vi "Read-Humidity.vi"(7 "Slave Address (7-bit)":u8 format="%x", 8 "error in (no error)":errorcluster, 9 "T_fine":dbl, 10 "Comp Coeffs":T1 {"dig_H6" format="%0d"; "dig_H5" format="%0d"; "dig_H4" format="%0d"; "dig_H3" format="%0d"; "dig_H2" format="%0d"; "dig_H1" format="%0d"; "dig_P9" format="%0d"; "dig_P8" format="%0d"; "dig_P7" format="%0d"; "dig_P6" format="%0d"; "dig_P5" format="%0d"; "dig_P4" format="%0d"; "dig_P3" format="%0d"; "dig_P2" format="%0d"; "dig_P1" format="%0d"; "dig_T3" format="%0d"; "dig_T2" format="%0d"; "dig_T1" format="%0d"}, 11 "I2C Ref In":T2) -> (0 "error out":errorcluster, 3 "I2C Ref Out":T2={"myRIO Reference"={"myRIO Model"=enum."Unknown", "myRIO Hardware Reference"={"Generic FPGA Reference"=refnum, "Allow multiple opens"=FALSE}}, "I2C Channels Enum"=enum."Not Connected", "I2C Configuration"={"I2C Transfer Rate"=enum."Fast mode (400 kbps)"}}, 4 "ADC RAW HUMIDITY":u32, 5 "Bytes Read":u8[](array[numeric]), 6 "Humidity":dbl)   [LabVIEW 2015]
uses:
  <vilib>/myRIO/Instrument Drivers/Onboard IO/I2C/typedefs/I2C Reference.ctl
  <vilib>/myRIO/Common/Instrument Driver Framework/Utilities/typedefs/myRIO Generic Hardware Reference.ctl
  <vilib>/myRIO/Common/Instrument Driver Framework/Utilities/typedefs/Hardware Version Enum.ctl
  <vilib>/myRIO/Common/Instrument Driver Framework/Utilities/typedefs/myRIO v1.0 Reference.ctl
  <vilib>/myRIO/Common/Instrument Driver Framework/Utilities/typedefs/Generic FPGA Reference.ctl
  <vilib>/myRIO/Common/Instrument Driver Framework/myRIO v1.0/I2C/typedefs/I2C Channels Enum.ctl
  <vilib>/myRIO/Instrument Drivers/Onboard IO/I2C/typedefs/I2C Configuration.ctl
  <vilib>/myRIO/Instrument Drivers/Onboard IO/I2C/typedefs/I2C Transfer Rate.ctl
  calib_data.ctl
  <vilib>/Utility/error.llb/Error Cluster From Error Code.vi
  <vilib>/myRIO/Common/Instrument Driver Framework/myRIO v1.0/I2C/vis/myRIO v1.0 Write I2C.vi
  <vilib>/myRIO/Common/Instrument Driver Framework/myRIO v1.0/I2C/vis/myRIO v1.0 Read I2C.vi
  <vilib>/myRIO/Instrument Drivers/Onboard IO/I2C/I2C.lvlib
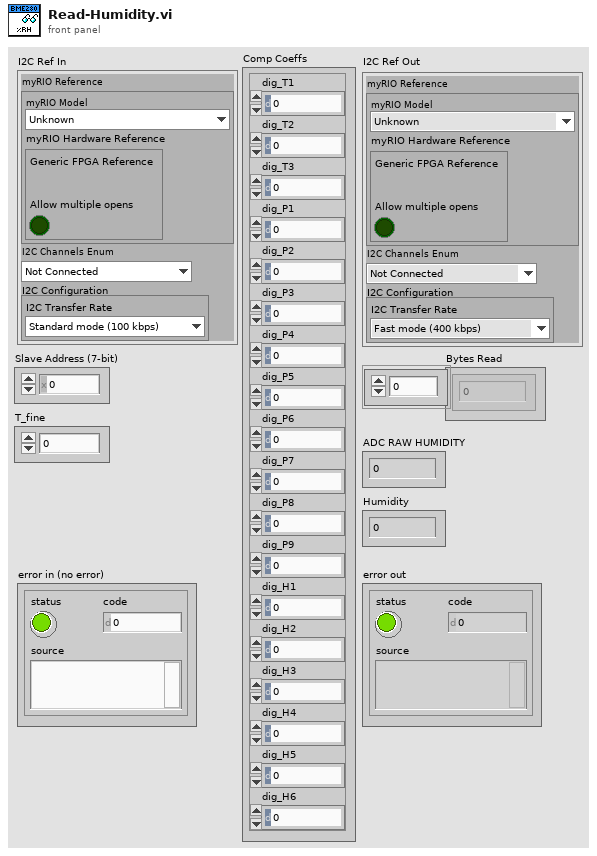
[diagram p1: front panel]
types:
  T1 = typedef "calib_data.ctl" = cluster{"dig_T1":u16, "dig_T2":i16, "dig_T3":i16, "dig_P1":u16, "dig_P2":i16, "dig_P3":i16, "dig_P4":i16, "dig_P5":i16, "dig_P6":i16, "dig_P7":i16, "dig_P8":i16, "dig_P9":i16, "dig_H1":u8, "dig_H2":i16, "dig_H3":u8, "dig_H4":i16, "dig_H5":i16, "dig_H6":i8}
  T2 = typedef "I2C.lvlib/I2C Reference.ctl" = cluster{"myRIO Reference":T3, "I2C Channels Enum":T7, "I2C Configuration":T8}
  T3 = typedef "myRIO Generic Hardware Reference.ctl" = cluster{"myRIO Model":T4, "myRIO Hardware Reference":T5}
  T4 = typedef "Hardware Version Enum.ctl" = enum16{"Unknown", "myRIO-1900", "myRIO-1950", "roboRIO"}
  T5 = typedef "myRIO v1.0 Reference.ctl" = cluster{"Generic FPGA Reference":T6, "Allow multiple opens":bool}
  T6 = typedef "Generic FPGA Reference.ctl" = refnum<k20>
  T7 = typedef "I2C Channels Enum.ctl" = enum16{"Not Connected", "A/I2C", "B/I2C", "I2C/I2C"}
  T8 = typedef "I2C.lvlib/I2C Configuration.ctl" = cluster{"I2C Transfer Rate":T9}
  T9 = typedef "I2C.lvlib/I2C Transfer Rate.ctl" = enum16{"Standard mode (100 kbps)", "Fast mode (400 kbps)"}
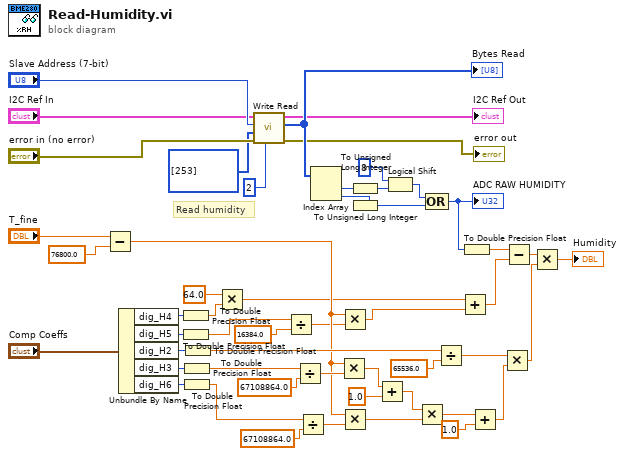
[diagram p0: block diagram]
diagram:
  # "Read humidity"
  n1 = Subtract(x="T_fine", y=76800.0) -> (x-y=w6:dbl)
  n2 = Unbundle By Name("Comp Coeffs") -> ("dig_H4"=w12:i16, "dig_H5"=w13:i16, "dig_H2"=w31:i16, "dig_H3"=w30:u8, "dig_H6"=w29:i8)
  n3 = To Double Precision Float(number=w12) -> (double precision float=w11:dbl)
  n4 = To Double Precision Float(number=w13) -> (double precision float=w8:dbl)
  n5 = To Double Precision Float(number=w30) -> (double precision float=w28:dbl)
  n6 = To Double Precision Float(number=w29) -> (double precision float=w23:dbl)
  n7 = To Double Precision Float(number=w31) -> (double precision float=w35:dbl)
  n8 = Multiply(x=64.0, y=w11) -> (x*y=w4:dbl)
  n9 = call <vilib>:"Write Read.vi"("Byte Count"=u32 2, "error in (no error)"="error in (no error)", "Bytes to Write"=u8[] [253], "Slave Address (7-bit)"="Slave Address (7-bit)", "I2C Ref In"="I2C Ref In") -> ("error out"=→"error out":errorcluster, "Bytes Read"=w45:u8[], "I2C Ref Out"=→"I2C Ref Out":T2)  [unwired: 3 in]
  "Bytes Read" <- w45
  n10 = Divide(x=w8, y=16384.0) -> (x/y=w5:dbl)
  n11 = Divide(x=w28, y=67108864.0) -> (x/y=w26:dbl)
  n12 = Divide(x=w23, y=67108864.0) -> (x/y=w21:dbl)
  n13 = Index Array(array=w45) -> (element #1=w44:u8, element #2=w48:u8)  [unwired: 2 in]
  n14 = Multiply(x=w6, y=w26) -> (x*y=w25:dbl)
  n15 = Multiply(x=w6, y=w5) -> (x*y=w3:dbl)
  n16 = Multiply(x=w6, y=w21) -> (x*y=w20:dbl)
  n17 = To Unsigned Long Integer(number=w44) -> (unsigned 32bit integer=w41:u32)
  n18 = To Unsigned Long Integer(number=w48) -> (unsigned 32bit integer=w49:u32)
  n19 = Add(x=w25, y=1.0) -> (x+y=w22:dbl)
  n20 = Logical Shift(y=u8 8 ("x"), x=w41) -> (x << y=w43:u32)
  n21 = Multiply(x=w22, y=w20) -> (x*y=w19:dbl)
  n22 = Compound Arithmetic op=OR(w43, w49) -> (w36:u32)
  "ADC RAW HUMIDITY" <- w36
  n23 = Divide(x=w35, y=65536.0) -> (x/y=w33:dbl)
  n24 = Add(x=w4, y=w3) -> (x+y=w9:dbl)
  n25 = To Double Precision Float(number=w36) -> (double precision float=w16:dbl)
  n26 = Add(x=w19, y=1.0) -> (x+y=w17:dbl)
  n27 = Multiply(x=w33, y=w17) -> (x*y=w15:dbl)
  n28 = Subtract(x=w16, y=w9) -> (x-y=w14:dbl)
  n29 = Multiply(x=w14, y=w15) -> (x*y=→"Humidity":dbl)
